vi "Initialize Local Reference.vi"(8 "error in (no error)":errorcluster, 10 "This VI":refnum<vi>, 11 "CIF_UI in":refnum<class "CIF_UI.lvclass">) -> (0 "error out":errorcluster, 3 "CIF_UI out":refnum<class "CIF_UI.lvclass">)   [LabVIEW 2021, in "CIF_UI.lvclass"]
uses:
  CIF_UI.lvclass
  CIF_UI.lvclass/CIF_UI.ctl
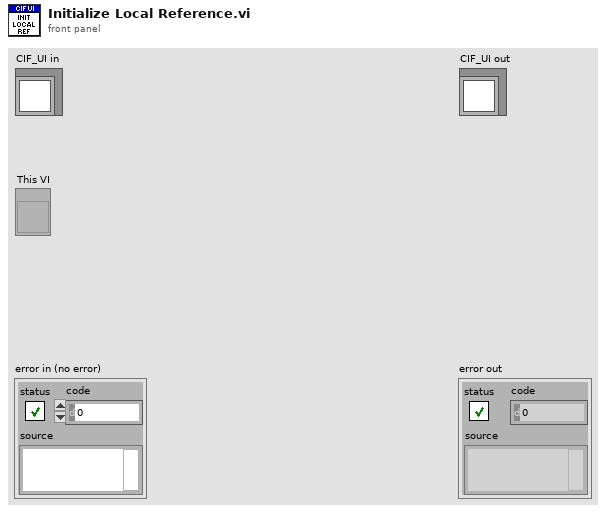
[diagram p1: front panel]
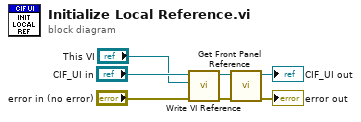
[diagram p0: block diagram]
diagram:
  n1 = call "Write VI Reference.vi"("error in (no error)"="error in (no error)", "VI Reference"="This VI", "CIF_UI in"="CIF_UI in") -> ("error out"=w3:errorcluster, "CIF_UI out"=w6:refnum<class "CIF_UI.lvclass">)  [unwired: 7 in]
  n2 = call "Get Front Panel Reference.vi"("error in (no error)"=w3, "CIF_UI in"=w6) -> ("error out"=→"error out":errorcluster, "CIF_UI out"=→"CIF_UI out":refnum<class "CIF_UI.lvclass">)  [unwired: 8 in]
